vi "getversion.vi"(8 "error in (no error)":errorcluster, 11 "MSCU":refnum<class "MSCU.lvclass">) -> (0 "error out":errorcluster, 1 "Revision":string, 2 "Version":string, 3 "MSCU":refnum<class "MSCU.lvclass">)   [LabVIEW 2019, in "MSCU.lvclass"]
uses:
  MSCU.lvclass
  MSCU.lvclass/MSCU.ctl
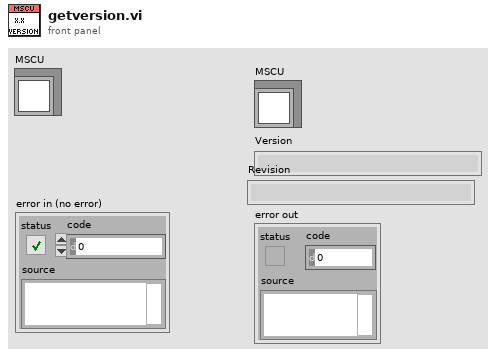
[diagram p1: front panel]
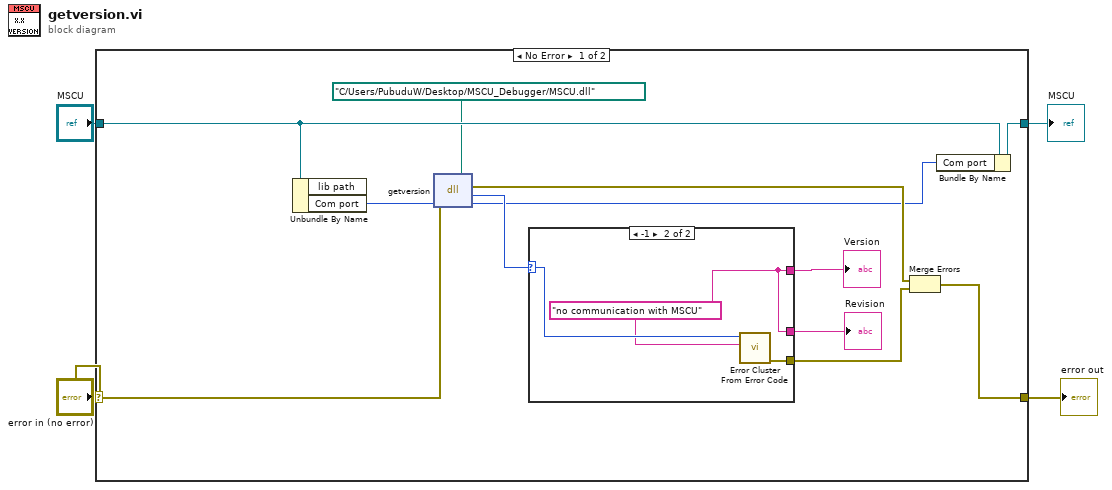
[diagram p0: block diagram]
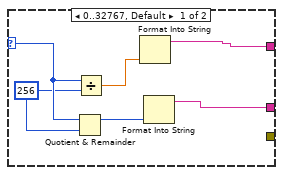
[diagram p2: hidden frame]
diagram:
  n1 = case shown="No Error" "error in (no error)" {
    selector: "error in (no error)" -> [w9 w26]
    tunnel: [w13 w27] -> w4
    tunnel: "MSCU" -> [w10 w27]
    tunnel: [w6 w26] -> w1
    frame No Error {
      n2 = Unbundle By Name(w10) -> ("Com port"=w11:i32)  [unwired: 1 out]
      n3 = dll-call lib="C:/Program Files (x86)/Nanonis/SPM Controller/data/MSCU.dll" fn="getversion"(path in=path "C:/Users/PubuduW/Desktop/MSCU_Debugger/MSCU.dll", error in=w9, "Comport"=w11) -> (error out=w14:errorcluster, "return type"=w16:i32, "Comport"=w12:i32)  [unwired: 1 in, 1 out]
      n4 = case shown="-1" w16 {
        selector: w16 -> [w22 w25]
        tunnel: [w19 w23] -> w15
        tunnel: [_ w24] -> w8
        tunnel: [w17 w23] -> w7
        frame 0..32767, Default {
          w21 = 256 ("y")
          n5 = Quotient & Remainder(x=w22, y=w21) -> (x-y*floor(x/y)=w18:i32)  [unwired: 1 out]
          n6 = Divide(x=w22, y=w21) -> (x/y=w20:dbl)
          n7 = Format Into String(w20) -> (resulting string=w19:string)  [unwired: 3 in, 1 out]
          n8 = Format Into String(w18) -> (resulting string=w17:string)  [unwired: 3 in, 1 out]
        }
        frame -1 {
          w23 = "no communication with MSCU"
          n9 = call <vilib>:"Error Cluster From Error Code.vi"("error message (\"\")"=w23, "error code (0)"=w25) -> ("error out"=w24:errorcluster)  [unwired: 7 in]
        }
      }
      "Version" <- w15
      "Revision" <- w7
      n10 = Merge Errors(w14, w8) -> (w6:errorcluster)
      n11 = Bundle By Name(cluster=w10, "Com port"=w12) -> (w13:refnum<class "MSCU.lvclass">)
    }
    frame Error {
    }
  }
  "MSCU" <- w4
  "error out" <- w1
